vi "Testing new Qs.vi"() -> ()   [LabVIEW 2021, in "Q Async.lvlib"]
uses:
  Q Async.lvlib
  Q Loop.vi
panel:
  in  "Numeric":i32=4
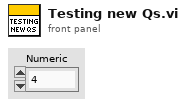
[diagram p1: front panel]
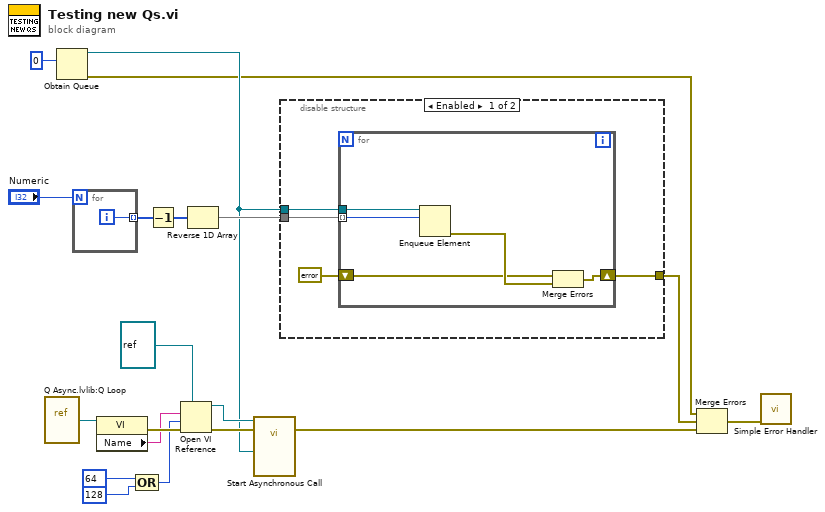
[diagram p0: block diagram]
diagram:
  n1 = vi-ref "Q Async.lvlib:Q Loop.vi"() -> (w11:refnum<vi>)
  n2 = Obtain Queue(element data type=0) -> (queue out=w2:refnum<queue>, error out=w1:errorcluster)  [unwired: 4 in, 1 out]
  n3 = for {
    N: "Numeric" -> [_]
    tunnel: [w20] -> w18 mode=indexing
    i -> [w20]
  }
  n4 = property class="VI"(reference=w11) -> (error out=w10:errorcluster, "Name"=w9:string)  [unwired: 1 in, 1 out]
  n5 = Compound Arithmetic op=OR(64 ("options"), 128 ("options")) -> (w6:i32)
  n6 = Decrement(x=w18) -> (x-1=w19:i32[])
  n7 = Open VI Reference(type specifier VI Refnum (for type only)=refnum<vi> refnum, vi path=w9, options=w6, error in (no error)=w10) -> (vi reference=w4:refnum<vi>, error out=w5:errorcluster)  [unwired: 2 in]
  n8 = Reverse 1D Array(array=w19) -> (reversed array=w15:i32[])
  n9 = call-by-ref "Start Asynchronous Call"(reference=w4, error in=w5, "Q"=w2) -> (error out=w3:errorcluster)  [unwired: 11 in, 1 out]
  n10 = disable-structure shown="Enabled" {
    disable-tunnel: w15 -> [w24 _]
    disable-tunnel: [w22 _] -> w14
    disable-tunnel: w2 -> [w21 _]
    frame Enabled {
      n11 = for {
        tunnel: w21 -> [w25]
        tunnel: w24 -> [w29] mode=indexing
        shift-right: [w27] -> w22
        shift-left: errorcluster {"status"=FALSE, "code"=0, "source"=""} ("error out") -> [w26]
        n12 = Enqueue Element(queue=w25, element=w29) -> (error out=w28:errorcluster)  [unwired: 2 in, 2 out]
        n13 = Merge Errors(w26, w28) -> (w27:errorcluster)
      }
    }
    frame Disabled {
    }
  }
  n14 = Merge Errors(w1, w14, w3) -> (w13:errorcluster)
  n15 = call <vilib>:"Simple Error Handler.vi"("error in (no error)"=w13) -> ()  [unwired: 4 in, 5 out]
